vi "Save(X,Y,dX,dY)_in_Array-1.vi"(2 "Array for Replacement IN":dbl[](array[numeric]), 3 "Starting Position":i32, 4 "dY":dbl, 5 "dX":dbl, 6 "Y":dbl, 7 "X":dbl) -> (0 "Finish Position":i32, 1 "Array for Replacement OUT":dbl[](array[numeric]))   [LabVIEW 2013]
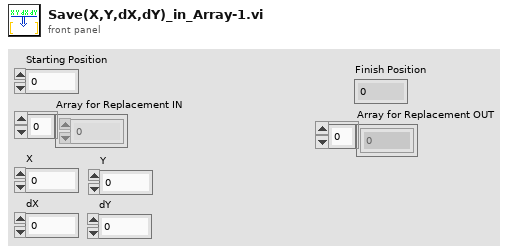
[diagram p1: front panel]
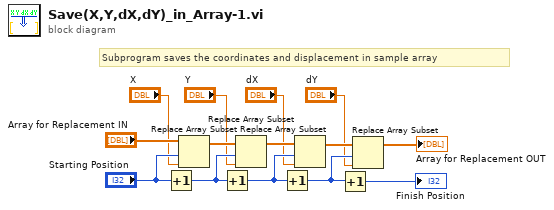
[diagram p0: block diagram]
diagram:
  # "Subprogram saves the coordinates and displacement in sample array"
  n1 = Increment(x="Starting Position") -> (x+1=w13:i32)
  n2 = Replace Array Subset(array="Array for Replacement IN", new element="X", index="Starting Position") -> (w14:dbl[])
  n3 = Increment(x=w13) -> (x+1=w11:i32)
  n4 = Replace Array Subset(array=w14, new element="Y", index=w13) -> (w12:dbl[])
  n5 = Increment(x=w11) -> (x+1=w10:i32)
  n6 = Replace Array Subset(array=w12, new element="dX", index=w11) -> (w9:dbl[])
  n7 = Increment(x=w10) -> (x+1=→"Finish Position":i32)
  n8 = Replace Array Subset(array=w9, new element="dY", index=w10) -> (→"Array for Replacement OUT":dbl[])
